vi "Lin Daten laden speichern Allgemein.vi"(9 "Index & MB":T1, 11 "Aktionen":T2) -> (1 "Index & MB":T1)   [LabVIEW 2020, in "Linearisierung v2.lvlib" / "Gasteiler.lvlib"]
uses:
  Gasteiler.lvlib
  Lin Daten verwalten Aktionen.ctl
  Index & MB.ctl
  <vilib>/Utility/config.llb/Write Key (String).vi
  <vilib>/Utility/config.llb/Read Key (String).vi
  <vilib>/Utility/config.llb/NI_LVConfig.lvlib
  Allgemein/allgemeine Sub-VIs.lvlib
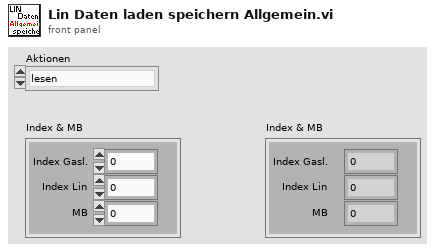
[diagram p1: front panel]
types:
  T1 = typedef "Linearisierung v2.lvlib/Gasteiler.lvlib/Index & MB.ctl" = cluster{"Index Gasl.":u16, "Index Lin":u16, "MB":u16}
  T2 = typedef "Linearisierung v2.lvlib/Gasteiler.lvlib/Lin Daten verwalten Aktionen.ctl" = enum16{"lesen", "speichern", "laden", "Lin Daten schr.", "Stufen Tabelle", "Lin Name AK", "Lin Pfad AK", "Umkehren"}
  T3 = typedef "NI_LVConfig.lvlib/Config Data RefNum.ctl" = refnum<k1>
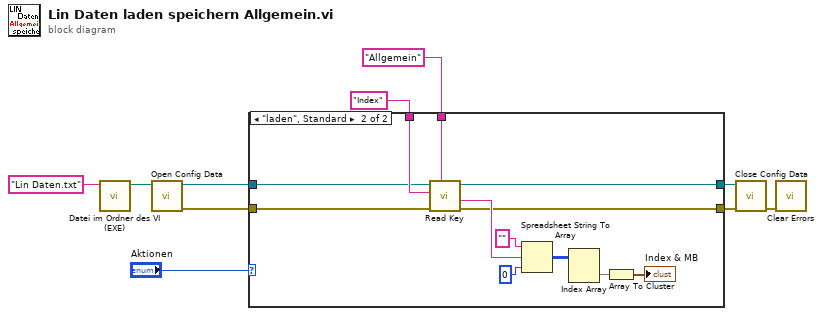
[diagram p0: block diagram]
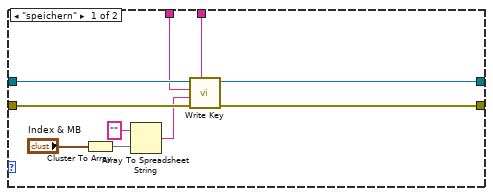
[diagram p2: hidden frame]
diagram:
  n1 = call "Datei im Ordner des VI (EXE).vi"("Dateiname"="Lin Daten.txt") -> ("Dateipfad im Ordner des Haupt-VIs"=w10:path)  [unwired: 8 in, 2 out]
  n2 = call <vilib>:"Open Config Data.vi"("configuration file path"=w10) -> ("error out"=w7:errorcluster, "refnum"=w8:T3)  [unwired: 8 in, 1 out]
  n3 = case shown="\"laden\", Standard" "Aktionen" {
    tunnel: w8 -> [w20 w29]
    tunnel: w7 -> [w19 w30]
    tunnel: [w12 w21] -> w6
    tunnel: [w11 w22] -> w5
    tunnel: "Index" ("key") -> [w18 w31]
    tunnel: "Allgemein" ("Dezimal-Integer-String") -> [w17 w32]
    frame "speichern" {
      n4 = Cluster To Array(cluster="Index & MB") -> (array=w16:u16[])
      n5 = Array To Spreadsheet String(array=w16, 3:"" ("Format-String")) -> (spreadsheet string=w13:string)  [unwired: 1 in]
      n6 = call-poly <vilib>:"Write Key.vi"("section"=w17, "error in (no error)"=w19, "value"=w13, "key"=w18, "refnum"=w20) -> ("error out"=w11:errorcluster, "refnum out"=w12:T3)  [unwired: 4 in, 1 out]
    }
    frame "laden", Default {
      n7 = call-poly <vilib>:"Read Key.vi"("section"=w32, "error in (no error)"=w30, "key"=w31, "refnum"=w29) -> ("error out"=w22:errorcluster, "value"=w27:string, "refnum out"=w21:T3)  [unwired: 4 in, 1 out]
      n8 = Spreadsheet String To Array(format string="" ("Format-String"), spreadsheet string=w27, array type (2D Dbl)=u16 0) -> (array=w25:u16[][])  [unwired: 1 in]
      n9 = Index Array(array=w25) -> (element=w24:u16[])  [unwired: 2 in]
      n10 = Array To Cluster(array=w24) -> (cluster=→"Index & MB":cluster{"[0]":u16, "[1]":u16, "[2]":u16})
    }
  }
  n11 = call <vilib>:"Close Config Data.vi"("error in (no error)"=w5, "refnum"=w6) -> ("error out"=w2:errorcluster)  [unwired: 8 in, 1 out]
  n12 = call <vilib>:"Clear Errors.vi"("error in (no error)"=w2) -> ()  [unwired: 5 in, 2 out]
